vi "WebView2 Viewer.vi"(2 "ProjectRef":refnum<vi>, 4 "Extra Scripts":string, 5 "FileDependency In":map{path, T1}(c390), 6 "Options":string, 7 "OpenWebBrowser(False)":bool, 8 "error in":errorcluster, 9 "Embedd VISJS Librarya in HTMl File(False)":bool, 10 "HTMLFilePath":path, 11 "LibraryDependency":map{path, T3}(c390)) -> (0 "error out":errorcluster, 3 "HTMLFileContent":string)   [LabVIEW 2020, in "WebView2-Viewer.lvlib"] (continued)
selfReference property instead. The selfReference can be set like thise selfReference:{size:30, angle:Math.PI / 4}\"),g.selfReference.size=t.selfReferenceSize)}}]),g}(),FR=function(){function g(t,A,e){var C,I=this;cn(this,g),this.body=t,this.images=A,this.groups=e,this.body.functions.createEdge=je(C=this.create).call(C,this),this.edgesListeners={add:function(g,t){I.add(t.items)},update:function(g,t){I.update(t.items)},remove:function(g,t){I.remove(t.items)}},this.options={},this.defaultOptions={arrows:{to:{enabled:!1,scaleFactor:1,type:\"arrow\"},middle:{enabled:!1,scaleFactor:1,type:\"arrow\"},from:{enabled:!1,scaleFactor:1,type:\"arrow\"}},endPointOffset:{from:0,to:0},arrowStrikethrough:!0,color:{color:\"#848484\",highlight:\"#848484\",hover:\"#848484\",inherit:\"from\",opacity:1},dashes:!1,font:{color:\"#343434\",size:14,face:\"arial\",background:\"none\",strokeWidth:2,strokeColor:\"#ffffff\",align:\"horizontal\",multi:!1,vadjust:0,bold:{mod:\"bold\"},boldital:{mod:\"bold italic\"},ital:{mod:\"italic\"},mono:{mod:\"\",size:15,face:\"courier new\",vadjust:2}},hidden:!1,hoverWidth:1.5,label:void 0,labelHighlightBold:!0,length:void 0,physics:!0,scaling:{min:1,max:15,label:{enabled:!0,min:14,max:30,maxVisible:30,drawThreshold:5},customScalingFunction:function(g,t,A,e){if(t===g)return.5;var C=1/(t-g);return Math.max(0,(e-g)*C)}},selectionWidth:1.5,selfReference:{size:20,angle:Math.PI/4,renderBehindTheNode:!0},shadow:{enabled:!1,color:\"rgba(0,0,0,0.5)\",size:10,x:5,y:5},background:{enabled:!1,color:\"rgba(111,111,111,1)\",size:10,dashes:!1},smooth:{enabled:!0,type:\"dynamic\",forceDirection:\"none\",roundness:.5},title:void 0,width:1,value:void 0},qf(this.options,this.defaultOptions),this.bindEventListeners()}return kd(g,[{key:\"bindEventListeners\",value:function(){var g,t,A=this;this.body.emitter.on(\"_forceDisableDynamicCurves\",(function(g){var t=!(arguments.length>1&&void 0!==arguments[1])||arguments[1];\"dynamic\"===g&&(g=\"continuous\");var e=!1;for(var C in A.body.edges)if(Object.prototype.hasOwnProperty.call(A.body.edges,C)){var I=A.body.edges[C],i=A.body.data.edges.get(C);if(null!=i){var o=i.smooth;void 0!==o&&!0===o.enabled&&\"dynamic\"===o.type&&(void 0===g?I.setOptions({smooth:!1}):I.setOptions({smooth:{type:g}}),e=!0)}}!0===t&&!0===e&&A.body.emitter.emit(\"_dataChanged\")})),this.body.emitter.on(\"_dataUpdated\",(function(){A.reconnectEdges()})),this.body.emitter.on(\"refreshEdges\",je(g=this.refresh).call(g,this)),this.body.emitter.on(\"refresh\",je(t=this.refresh).call(t,this)),this.body.emitter.on(\"destroy\",(function(){tv(A.edgesListeners,(function(g,t){A.body.data.edges&&A.body.data.edges.off(t,g)})),delete A.body.functions.createEdge,delete A.edgesListeners.add,delete A.edgesListeners.update,delete A.edgesListeners.remove,delete A.edgesListeners}))}},{key:\"setOptions\",value:function(g){if(void 0!==g){ZR.parseOptions(this.options,g,!0,this.defaultOptions,!0);var t=!1;if(void 0!==g.smooth)for(var A in this.body.edges)Object.prototype.hasOwnProperty.call(this.body.edges,A)&&(t=this.body.edges[A].updateEdgeType()||t);if(void 0!==g.font)for(var e in this.body.edges)Object.prototype.hasOwnProperty.call(this.body.edges,e)&&this.body.edges[e].updateLabelModule();void 0===g.hidden&&void 0===g.physics&&!0!==t||this.body.emitter.emit(\"_dataChanged\")}}},{key:\"setData\",value:function(g){var t=this,A=arguments.length>1&&void 0!==arguments[1]&&arguments[1],e=this.body.data.edges;if(kD(\"id\",g))this.body.data.edges=g;else if(Rh(g))this.body.data.edges=new mD,this.body.data.edges.add(g);else{if(g)throw new TypeError(\"Array or DataSet expected\");this.body.data.edges=new mD}if(e&&tv(this.edgesListeners,(function(g,t){e.off(t,g)})),this.body.edges={},this.body.data.edges){tv(this.edgesListeners,(function(g,A){t.body.data.edges.on(A,g)}));var C=this.body.data.edges.getIds();this.add(C,!0)}this.body.emitter.emit(\"_adjustEdgesForHierarchicalLayout\"),!1===A&&this.body.emitter.emit(\"_dataChanged\")}},{key:\"add\",value:function(g){for(var t=arguments.length>1&&void 0!==arguments[1]&&arguments[1],A=this.body.edges,e=this.body.data.edges,C=0;C<g.length;C++){var I=g[C],i=A[I];i&&i.disconnect();var o=e.get(I,{showInternalIds:!0});A[I]=this.create(o)}this.body.emitter.emit(\"_adjustEdgesForHierarchicalLayout\"),!1===t&&this.body.emitter.emit(\"_dataChanged\")}},{key:\"update\",value:function(g){for(var t=this.body.edges,A=this.body.data.edges,e=!1,C=0;C<g.length;C++){var I=g[C],i=A.get(I),o=t[I];void 0!==o?(o.disconnect(),e=o.setOptions(i)||e,o.connect()):(this.body.edges[I]=this.create(i),e=!0)}!0===e?(this.body.emitter.emit(\"_adjustEdgesForHierarchicalLayout\"),this.body.emitter.emit(\"_dataChanged\")):this.body.emitter.emit(\"_dataUpdated\")}},{key:\"remove\",value:function(g){var t=!(arguments.length>1&&void 0!==arguments[1])||arguments[1];if(0!==g.length){var A=this.body.edges;tv(g,(function(g){var t=A[g];void 0!==t&&t.remove()})),t&&this.body.emitter.emit(\"_dataChanged\")}}},{key:\"refresh\",value:function(){var g=this;tv(this.body.edges,(function(t,A){var e=g.body.data.edges.get(A);void 0!==e&&t.setOptions(e)}))}},{key:\"create\",value:function(g){return new ZR(g,this.body,this.images,this.options,this.defaultOptions)}},{key:\"reconnectEdges\",value:function(){var g,t=this.body.nodes,A=this.body.edges;for(g in t)Object.prototype.hasOwnProperty.call(t,g)&&(t[g].edges=[]);for(g in A)if(Object.prototype.hasOwnProperty.call(A,g)){var e=A[g];e.from=null,e.to=null,e.connect()}}},{key:\"getConnectedNodes\",value:function(g){var t=[];if(void 0!==this.body.edges[g]){var A=this.body.edges[g];void 0!==A.fromId&&t.push(A.fromId),void 0!==A.toId&&t.push(A.toId)}return t}},{key:\"_updateState\",value:function(){this._addMissingEdges(),this._removeInvalidEdges()}},{key:\"_removeInvalidEdges\",value:function(){var g=this,t=[];tv(this.body.edges,(function(A,e){var C=g.body.nodes[A.toId],I=g.body.nodes[A.fromId];void 0!==C&&!0===C.isCluster||void 0!==I&&!0===I.isCluster||void 0!==C&&void 0!==I||t.push(e)})),this.remove(t,!1)}},{key:\"_addMissingEdges\",value:function(){var g=this.body.data.edges;if(null!=g){var t=this.body.edges,A=[];Cl(g).call(g,(function(g,e){void 0===t[e]&&A.push(e)})),this.add(A,!0)}}}]),g}(),GR=function(){function g(t,A,e){cn(this,g),this.body=t,this.physicsBody=A,this.barnesHutTree,this.setOptions(e),this._rng=Ff(\"BARNES HUT SOLVER\")}return kd(g,[{key:\"setOptions\",value:function(g){this.options=g,this.thetaInversed=1/this.options.theta,this.overlapAvoidanceFactor=1-Math.max(0,Math.min(1,this.options.avoidOverlap))}},{key:\"solve\",value:function(){if(0!==this.options.gravitationalConstant&&this.physicsBody.physicsNodeIndices.length>0){var g,t=this.body.nodes,A=this.physicsBody.physicsNodeIndices,e=A.length,C=this._formBarnesHutTree(t,A);this.barnesHutTree=C;for(var I=0;I<e;I++)(g=t[A[I]]).options.mass>0&&this._getForceContributions(C.root,g)}}},{key:\"_getForceContributions\",value:function(g,t){this._getForceContribution(g.children.NW,t),this._getForceContribution(g.children.NE,t),this._getForceContribution(g.children.SW,t),this._getForceContribution(g.children.SE,t)}},{key:\"_getForceContribution\",value:function(g,t){if(g.childrenCount>0){var A=g.centerOfMass.x-t.x,e=g.centerOfMass.y-t.y,C=Math.sqrt(A*A+e*e);C*g.calcSize>this.thetaInversed?this._calculateForces(C,A,e,t,g):4===g.childrenCount?this._getForceContributions(g,t):g.children.data.id!=t.id&&this._calculateForces(C,A,e,t,g)}}},{key:\"_calculateForces\",value:function(g,t,A,e,C){0===g&&(t=g=.1),this.overlapAvoidanceFactor<1&&e.shape.radius&&(g=Math.max(.1+this.overlapAvoidanceFactor*e.shape.radius,g-e.shape.radius));var I=this.options.gravitationalConstant*C.mass*e.options.mass/Math.pow(g,3),i=t*I,o=A*I;this.physicsBody.forces[e.id].x+=i,this.physicsBody.forces[e.id].y+=o}},{key:\"_formBarnesHutTree\",value:function(g,t){for(var A,e=t.length,C=g[t[0]].x,I=g[t[0]].y,i=g[t[0]].x,o=g[t[0]].y,n=1;n<e;n++){var r=g[t[n]],s=r.x,a=r.y;r.options.mass>0&&(s<C&&(C=s),s>i&&(i=s),a<I&&(I=a),a>o&&(o=a))}var d=Math.abs(i-C)-Math.abs(o-I);d>0?(I-=.5*d,o+=.5*d):(C+=.5*d,i-=.5*d);var h=Math.max(1e-5,Math.abs(i-C)),l=.5*h,c=.5*(C+i),u=.5*(I+o),p={root:{centerOfMass:{x:0,y:0},mass:0,range:{minX:c-l,maxX:c+l,minY:u-l,maxY:u+l},size:h,calcSize:1/h,children:{data:null},maxWidth:0,level:0,childrenCount:4}};this._splitBranch(p.root);for(var f=0;f<e;f++)(A=g[t[f]]).options.mass>0&&this._placeInTree(p.root,A);return p}},{key:\"_updateBranchMass\",value:function(g,t){var A=g.centerOfMass,e=g.mass+t.options.mass,C=1/e;A.x=A.x*g.mass+t.x*t.options.mass,A.x*=C,A.y=A.y*g.mass+t.y*t.options.mass,A.y*=C,g.mass=e;var I=Math.max(Math.max(t.height,t.radius),t.width);g.maxWidth=g.maxWidth<I?I:g.maxWidth}},{key:\"_placeInTree\",value:function(g,t,A){1==A&&void 0!==A||this._updateBranchMass(g,t);var e,C=g.children.NW.range;e=C.maxX>t.x?C.maxY>t.y?\"NW\":\"SW\":C.maxY>t.y?\"NE\":\"SE\",this._placeInRegion(g,t,e)}},{key:\"_placeInRegion\",value:function(g,t,A){var e=g.children[A];switch(e.childrenCount){case 0:e.children.data=t,e.childrenCount=1,this._updateBranchMass(e,t);break;case 1:e.children.data.x===t.x&&e.children.data.y===t.y?(t.x+=this._rng(),t.y+=this._rng()):(this._splitBranch(e),this._placeInTree(e,t));break;case 4:this._placeInTree(e,t)}}},{key:\"_splitBranch\",value:function(g){var t=null;1===g.childrenCount&&(t=g.children.data,g.mass=0,g.centerOfMass.x=0,g.centerOfMass.y=0),g.childrenCount=4,g.children.data=null,this._insertRegion(g,\"NW\"),this._insertRegion(g,\"NE\"),this._insertRegion(g,\"SW\"),this._insertRegion(g,\"SE\"),null!=t&&this._placeInTree(g,t)}},{key:\"_insertRegion\",value:function(g,t){var A,e,C,I,i=.5*g.size;switch(t){case\"NW\":A=g.range.minX,e=g.range.minX+i,C=g.range.minY,I=g.range.minY+i;break;case\"NE\":A=g.range.minX+i,e=g.range.maxX,C=g.range.minY,I=g.range.minY+i;break;case\"SW\":A=g.range.minX,e=g.range.minX+i,C=g.range.minY+i,I=g.range.maxY;break;case\"SE\":A=g.range.minX+i,e=g.range.maxX,C=g.range.minY+i,I=g.range.maxY}g.children[t]={centerOfMass:{x:0,y:0},mass:0,range:{minX:A,maxX:e,minY:C,maxY:I},size:.5*g.size,calcSize:2*g.calcSize,children:{data:null},maxWidth:0,level:g.level+1,childrenCount:0}}},{key:\"_debug\",value:function(g,t){void 0!==this.barnesHutTree&&(g.lineWidth=1,this._drawBranch(this.barnesHutTree.root,g,t))}},{key:\"_drawBranch\",value:function(g,t,A){void 0===A&&(A=\"#FF0000\"),4===g.childrenCount&&(this._drawBranch(g.children.NW,t),this._drawBranch(g.children.NE,t),this._drawBranch(g.children.SE,t),this._drawBranch(g.children.SW,t)),t.strokeStyle=A,t.beginPath(),t.moveTo(g.range.minX,g.range.minY),t.lineTo(g.range.maxX,g.range.minY),t.stroke(),t.beginPath(),t.moveTo(g.range.maxX,g.range.minY),t.lineTo(g.range.maxX,g.range.maxY),t.stroke(),t.beginPath(),t.moveTo(g.range.maxX,g.range.maxY),t.lineTo(g.range.minX,g.range.maxY),t.stroke(),t.beginPath(),t.moveTo(g.range.minX,g.range.maxY),t.lineTo(g.range.minX,g.range.minY),t.stroke()}}]),g}(),jR=function(){function g(t,A,e){cn(this,g),this._rng=Ff(\"REPULSION SOLVER\"),this.body=t,this.physicsBody=A,this.setOptions(e)}return kd(g,[{key:\"setOptions\",value:function(g){this.options=g}},{key:\"solve\",value:function(){for(var g,t,A,e,C,I,i,o,n=this.body.nodes,r=this.physicsBody.physicsNodeIndices,s=this.physicsBody.forces,a=this.options.nodeDistance,d=-2/3/a,h=0;h<r.length-1;h++){i=n[r[h]];for(var l=h+1;l<r.length;l++)g=(o=n[r[l]]).x-i.x,t=o.y-i.y,0===(A=Math.sqrt(g*g+t*t))&&(g=A=.1*this._rng()),A<2*a&&(I=A<.5*a?1:d*A+1.3333333333333333,e=g*(I/=A),C=t*I,s[i.id].x-=e,s[i.id].y-=C,s[o.id].x+=e,s[o.id].y+=C)}}}]),g}(),LR=function(){function g(t,A,e){cn(this,g),this.body=t,this.physicsBody=A,this.setOptions(e)}return kd(g,[{key:\"setOptions\",value:function(g){this.options=g,this.overlapAvoidanceFactor=Math.max(0,Math.min(1,this.options.avoidOverlap||0))}},{key:\"solve\",value:function(){for(var g=this.body.nodes,t=this.physicsBody.physicsNodeIndices,A=this.physicsBody.forces,e=this.options.nodeDistance,C=0;C<t.length-1;C++)for(var I=g[t[C]],i=C+1;i<t.length;i++){var o=g[t[i]];if(I.level===o.level){var n=e+this.overlapAvoidanceFactor*((I.shape.radius||0)/2+(o.shape.radius||0)/2),r=o.x-I.x,s=o.y-I.y,a=Math.sqrt(r*r+s*s),d=void 0;d=a<n?-Math.pow(.05*a,2)+Math.pow(.05*n,2):0,0!==a&&(d/=a);var h=r*d,l=s*d;A[I.id].x-=h,A[I.id].y-=l,A[o.id].x+=h,A[o.id].y+=l}}}}]),g}(),VR=function(){function g(t,A,e){cn(this,g),this.body=t,this.physicsBody=A,this.setOptions(e)}return kd(g,[{key:\"setOptions\",value:function(g){this.options=g}},{key:\"solve\",value:function(){for(var g,t,A,e,C,I=this.physicsBody.physicsEdgeIndices,i=this.body.edges,o=0;o<I.length;o++)!0===(t=i[I[o]]).connected&&t.toId!==t.fromId&&void 0!==this.body.nodes[t.toId]&&void 0!==this.body.nodes[t.fromId]&&(void 0!==t.edgeType.via?(g=void 0===t.options.length?this.options.springLength:t.options.length,A=t.to,e=t.edgeType.via,C=t.from,this._calculateSpringForce(A,e,.5*g),this._calculateSpringForce(e,C,.5*g)):(g=void 0===t.options.length?1.5*this.options.springLength:t.options.length,this._calculateSpringForce(t.from,t.to,g)))}},{key:\"_calculateSpringForce\",value:function(g,t,A){var e=g.x-t.x,C=g.y-t.y,I=Math.max(Math.sqrt(e*e+C*C),.01),i=this.options.springConstant*(A-I)/I,o=e*i,n=C*i;void 0!==this.physicsBody.forces[g.id]&&(this.physicsBody.forces[g.id].x+=o,this.physicsBody.forces[g.id].y+=n),void 0!==this.physicsBody.forces[t.id]&&(this.physicsBody.forces[t.id].x-=o,this.physicsBody.forces[t.id].y-=n)}}]),g}(),YR=function(){function g(t,A,e){cn(this,g),this.body=t,this.physicsBody=A,this.setOptions(e)}return kd(g,[{key:\"setOptions\",value:function(g){this.options=g}},{key:\"solve\",value:function(){for(var g,t,A,e,C,I,i,o,n,r,s=this.body.edges,a=.5,d=this.physicsBody.physicsEdgeIndices,h=this.physicsBody.physicsNodeIndices,l=this.physicsBody.forces,c=0;c<h.length;c++){var u=h[c];l[u].springFx=0,l[u].springFy=0}for(var p=0;p<d.length;p++)!0===(t=s[d[p]]).connected&&(g=void 0===t.options.length?this.options.springLength:t.options.length,A=t.from.x-t.to.x,e=t.from.y-t.to.y,o=0===(o=Math.sqrt(A*A+e*e))?.01:o,C=A*(i=this.options.springConstant*(g-o)/o),I=e*i,t.to.level!=t.from.level?(void 0!==l[t.toId]&&(l[t.toId].springFx-=C,l[t.toId].springFy-=I),void 0!==l[t.fromId]&&(l[t.fromId].springFx+=C,l[t.fromId].springFy+=I)):(void 0!==l[t.toId]&&(l[t.toId].x-=a*C,l[t.toId].y-=a*I),void 0!==l[t.fromId]&&(l[t.fromId].x+=a*C,l[t.fromId].y+=a*I)));i=1;for(var f=0;f<h.length;f++){var v=h[f];n=Math.min(i,Math.max(-i,l[v].springFx)),r=Math.min(i,Math.max(-i,l[v].springFy)),l[v].x+=n,l[v].y+=r}for(var y=0,m=0,b=0;b<h.length;b++){var w=h[b];y+=l[w].x,m+=l[w].y}for(var k=y/h.length,x=m/h.length,E=0;E<h.length;E++){var O=h[E];l[O].x-=k,l[O].y-=x}}}]),g}(),WR=function(){function g(t,A,e){cn(this,g),this.body=t,this.physicsBody=A,this.setOptions(e)}return kd(g,[{key:\"setOptions\",value:function(g){this.options=g}},{key:\"solve\",value:function(){for(var g,t,A,e,C=this.body.nodes,I=this.physicsBody.physicsNodeIndices,i=this.physicsBody.forces,o=0;o<I.length;o++){g=-(e=C[I[o]]).x,t=-e.y,A=Math.sqrt(g*g+t*t),this._calculateForces(A,g,t,i,e)}}},{key:\"_calculateForces\",value:function(g,t,A,e,C){var I=0===g?0:this.options.centralGravity/g;e[C.id].x=t*I,e[C.id].y=A*I}}]),g}();function QR(g){var t=function(){if(\"undefined\"==typeof Reflect||!MT)return!1;if(MT.sham)return!1;if(\"function\"==typeof Proxy)return!0;try{return Boolean.prototype.valueOf.call(MT(Boolean,[],(function(){}))),!0}catch(g){return!1}}();return function(){var A,e=nb(g);if(t){var C=nb(this).constructor;A=MT(e,arguments,C)}else A=e.apply(this,arguments);return Ib(this,A)}}var UR=function(g){Cb(A,g);var t=QR(A);function A(g,e,C){var I;return cn(this,A),(I=t.call(this,g,e,C))._rng=Ff(\"FORCE ATLAS 2 BASED REPULSION SOLVER\"),I}return kd(A,[{key:\"_calculateForces\",value:function(g,t,A,e,C){0===g&&(t=g=.1*this._rng()),this.overlapAvoidanceFactor<1&&e.shape.radius&&(g=Math.max(.1+this.overlapAvoidanceFactor*e.shape.radius,g-e.shape.radius));var I=e.edges.length+1,i=this.options.gravitationalConstant*C.mass*e.options.mass*I/Math.pow(g,2),o=t*i,n=A*i;this.physicsBody.forces[e.id].x+=o,this.physicsBody.forces[e.id].y+=n}}]),A}(GR);function _R(g){var t=function(){if(\"undefined\"==typeof Reflect||!MT)return!1;if(MT.sham)return!1;if(\"function\"==typeof Proxy)return!0;try{return Boolean.prototype.valueOf.call(MT(Boolean,[],(function(){}))),!0}catch(g){return!1}}();return function(){var A,e=nb(g);if(t){var C=nb(this).constructor;A=MT(e,arguments,C)}else A=e.apply(this,arguments);return Ib(this,A)}}var KR=function(g){Cb(A,g);var t=_R(A);function A(g,e,C){return cn(this,A),t.call(this,g,e,C)}return kd(A,[{key:\"_calculateForces\",value:function(g,t,A,e,C){if(g>0){var I=C.edges.length+1,i=this.options.centralGravity*I*C.options.mass;e[C.id].x=t*i,e[C.id].y=A*i}}}]),A}(WR),HR=function(){function g(t){cn(this,g),this.body=t,this.physicsBody={physicsNodeIndices:[],physicsEdgeIndices:[],forces:{},velocities:{}},this.physicsEnabled=!0,this.simulationInterval=1e3/60,this.requiresTimeout=!0,this.previousStates={},this.referenceState={},this.freezeCache={},this.renderTimer=void 0,this.adaptiveTimestep=!1,this.adaptiveTimestepEnabled=!1,this.adaptiveCounter=0,this.adaptiveInterval=3,this.stabilized=!1,this.startedStabilization=!1,this.stabilizationIterations=0,this.ready=!1,this.options={},this.defaultOptions={enabled:!0,barnesHut:{theta:.5,gravitationalConstant:-2e3,centralGravity:.3,springLength:95,springConstant:.04,damping:.09,avoidOverlap:0},forceAtlas2Based:{theta:.5,gravitationalConstant:-50,centralGravity:.01,springConstant:.08,springLength:100,damping:.4,avoidOverlap:0},repulsion:{centralGravity:.2,springLength:200,springConstant:.05,nodeDistance:100,damping:.09,avoidOverlap:0},hierarchicalRepulsion:{centralGravity:0,springLength:100,springConstant:.01,nodeDistance:120,damping:.09},maxVelocity:50,minVelocity:.75,solver:\"barnesHut\",stabilization:{enabled:!0,iterations:1e3,updateInterval:50,onlyDynamicEdges:!1,fit:!0},timestep:.5,adaptiveTimestep:!0,wind:{x:0,y:0}},fe(this.options,this.defaultOptions),this.timestep=.5,this.layoutFailed=!1,this.bindEventListeners()}return kd(g,[{key:\"bindEventListeners\",value:function(){var g=this;this.body.emitter.on(\"initPhysics\",(function(){g.initPhysics()})),this.body.emitter.on(\"_layoutFailed\",(function(){g.layoutFailed=!0})),this.body.emitter.on(\"resetPhysics\",(function(){g.stopSimulation(),g.ready=!1})),this.body.emitter.on(\"disablePhysics\",(function(){g.physicsEnabled=!1,g.stopSimulation()})),this.body.emitter.on(\"restorePhysics\",(function(){g.setOptions(g.options),!0===g.ready&&g.startSimulation()})),this.body.emitter.on(\"startSimulation\",(function(){!0===g.ready&&g.startSimulation()})),this.body.emitter.on(\"stopSimulation\",(function(){g.stopSimulation()})),this.body.emitter.on(\"destroy\",(function(){g.stopSimulation(!1),g.body.emitter.off()})),this.body.emitter.on(\"_dataChanged\",(function(){g.updatePhysicsData()}))}},{key:\"setOptions\",value:function(g){if(void 0!==g)if(!1===g)this.options.enabled=!1,this.physicsEnabled=!1,this.stopSimulation();else if(!0===g)this.options.enabled=!0,this.physicsEnabled=!0,this.startSimulation();else{this.physicsEnabled=!0,Jf([\"stabilization\"],this.options,g),dv(this.options,g,\"stabilization\"),void 0===g.enabled&&(this.options.enabled=!0),!1===this.options.enabled&&(this.physicsEnabled=!1,this.stopSimulation());var t=this.options.wind;t&&((\"number\"!=typeof t.x||jm(t.x))&&(t.x=0),(\"number\"!=typeof t.y||jm(t.y))&&(t.y=0)),this.timestep=this.options.timestep}this.init()}},{key:\"init\",value:function(){var g;\"forceAtlas2Based\"===this.options.solver?(g=this.options.forceAtlas2Based,this.nodesSolver=new UR(this.body,this.physicsBody,g),this.edgesSolver=new VR(this.body,this.physicsBody,g),this.gravitySolver=new KR(this.body,this.physicsBody,g)):\"repulsion\"===this.options.solver?(g=this.options.repulsion,this.nodesSolver=new jR(this.body,this.physicsBody,g),this.edgesSolver=new VR(this.body,
